vi "Order Spectrum (Digital Tach).vi"(5 "window type":T3(ring)=enum."Hanning", 7 "dB On (T)":bool=TRUE, 8 "pulse/revolution (1)":i32=1, 9 "digital tach info":T1={"tacho counts"=[], "counter timebase [Hz]"=20000000.0, "counter task type"=enum."event counting", "counter digit (32)"=32}, 11 "scaled signal [EU]":waveform(dbl)={"t0"=timestamp(0 s since 1904-01-01), "dt"=0.0, "Y"=[]}) -> (0 "average speed [rpm]":dbl format="%.2f", 2 "unit label":string, 3 "order spectrum":T2 {"order 0" format="%.2p"; "delta order" format="%.2p"; "magnitude" format="%.2f"})   [LabVIEW 2017]
doc: "Computes the order spectrum (power vs. orders) for <B>scaled signal</B> and <B>digital tach info</B>."
uses:
  <vilib>/addons/Sound and Vibration/Order Analysis/Tach Process/SubVIs/digital tach info.ctl
  <vilib>/Analysis/baseanly.llb/Mean (DBL).vi
  <vilib>/addons/Sound and Vibration/Order Analysis/Backward Compatibility/OAT Sampled Power Spectrum (Single Channel).vi
  <vilib>/addons/Sound and Vibration/Order Analysis/Backward Compatibility/OAT Resample Waveform (Single Channel).vi
  <vilib>/Analysis/NI_AALBase.lvlib
  <vilib>/addons/Sound and Vibration/Order Analysis/Tach Process/SoundVib_TachProcess.lvlib
panel:
  # "Order Spectrum (Digital Tach)"
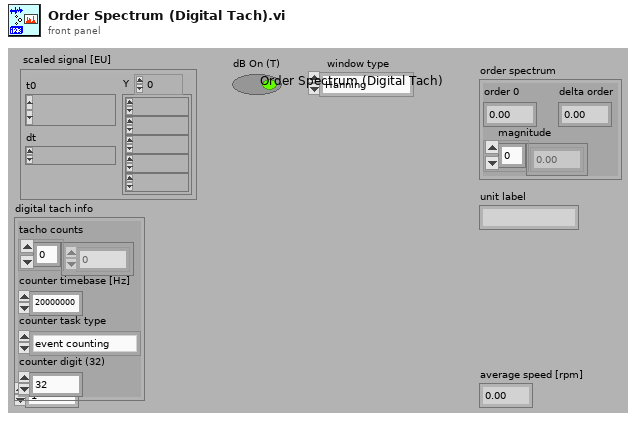
[diagram p1: front panel]
types:
  T1 = typedef "SoundVib_TachProcess.lvlib/digital tach info.ctl" = cluster{"tacho counts":i64[], "counter timebase [Hz]":dbl, "counter task type":enum16{"period measurement", "event counting"}, "counter digit (32)":i32}
  T2 = cluster{"order 0":dbl, "delta order":dbl, "magnitude":dbl[]}
  T3 = enum16{"None ", "Hanning", "Hamming", "Blackman-Harris", "Exact Blackman", "Blackman", "Flat Top", "4 Term B-Harris ", "7 Term B-Harris", "Low Sidelobe"}
  T4 = typedef "SoundVib_TachProcess.lvlib/speed profile.ctl" = cluster{"time [s]":dbl[], "speed [RPM]":dbl[]}
  T5 = cluster{"window type":enum16{"None ", "Hanning", "Hamming", "Blackman-Harris", "Exact Blackman", "Blackman", "Flat Top", "4 Term B-Harris ", "7 Term B-Harris", "Low Sidelobe"}, i32}
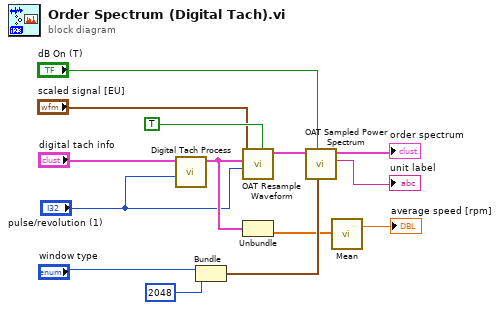
[diagram p0: block diagram]
diagram:
  n1 = call <vilib>:"Digital Tach Process.vi"("pulse/revolution (1)"="pulse/revolution (1)", "digital tach info"="digital tach info") -> ("speed profile"=w10:T4)  [unwired: 7 in, 2 out]
  n2 = Bundle("window type"="window type", 2048) -> (w11:T5)  [unwired: 1 in]
  n3 = call-poly <vilib>:"OAT Resample Waveform.vi"("reset? (True)"=TRUE ("reset? (TRUE)"), "pulse/revolution (1)"="pulse/revolution (1)", "speed profile"=w10, "scaled signal [EU]"="scaled signal [EU]") -> ("resampled signal"=w13:cluster{"r0":dbl, "dr":dbl, "Y":dbl[]})  [unwired: 4 in, 3 out]
  n4 = Unbundle(w10) -> ("speed [RPM]"=w9:dbl[])  [unwired: 1 out]
  n5 = call-poly <vilib>:"OAT Sampled Power Spectrum.vi"("window info"=w11, "dB On (T)"="dB On (T)", "resampled signal"=w13) -> ("unit label"=→"unit label":string, "order spectrum"=→"order spectrum":T2)  [unwired: 6 in, 1 out]
  n6 = call-poly <vilib>:"Mean.vi"("X"=w9) -> ("mean"=→"average speed [rpm]":dbl)  [unwired: 1 out]
